vi "Periodic Tasks.vi"(8 "error in":errorcluster) -> ()   [LabVIEW 2015]
doc: "This VI runs in parallel to other tasks. It can contain as many user-defined periodic loops as you need. These can carry out PID or other sorts of timed response."
uses:
  <vilib>/Rock Robotics/WPI/Solenoid/WPI_SolenoidValue.ctl
  <vilib>/Rock Robotics/WPI/Utilities/WPI_GetSetVariantRefNum.vi
  <vilib>/Rock Robotics/WPI/Solenoid/WPI_SolenoidSetEnum.vi
  Robot Global Data.vi
  Vision/Vision Global.vi
  <vilib>/addons/control/pid/pid.llb/PID (DBL).vi
  <vilib>/addons/control/pid/NI_PID_pid.lvlib
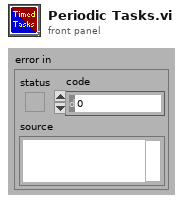
[diagram p1: front panel]
types:
  T1 = typedef "WPI_JoystickDevRef.ctl" = cluster{"Device":T2}
  T2 = typedef "WPI_JoystickDeviceEnum.ctl" = enum16{"USB 0", "USB 1", "USB 2", "USB 3", "USB 4", "USB 5"}
  T3 = typedef "WPI_MotorControlDeviceRef.ctl" = cluster{"DeviceStatus":errorcluster, "Type":T4, "PWM":cluster{"PWM Channel":T5, "DeadBand":T6}, "CAN":cluster{"Device Number":u8, "Control Mode":T7, "Semaphore":T8, "Max Vout":dbl, "TalonSRX Control Mode":T9}, "Invert":bool}
  T4 = typedef "WPI_MotorControlType.ctl" = enum16{"PWM", "CAN", "CANTalonSRX"}
  T5 = typedef "FPGA_DIOPWMChannel.ctl" = enum8{"PWM 0", "PWM 1", "PWM 2", "PWM 3", "PWM 4", "PWM 5", "PWM 6", "PWM 7", "PWM 8", "PWM 9", "PWM MXP 0", "PWM MXP 1", "PWM MXP 2", "PWM MXP 3", "PWM MXP 4", "PWM MXP 5", "PWM MXP 6", "PWM MXP 7", "PWM MXP 8", "PWM MXP 9", "Invalid"}
  T6 = typedef "WPI_PWMDeadband.ctl" = cluster{"Name":string, "maxPositivePwm":i32, "minPositivePwm":i32, "centerPwm":i32, "maxNegativePwm":i32, "minNegativePwm":i32, "angularRange":u16}
  T7 = typedef "WPI_CANJaguar_ControlMode.ctl" = enum8{"Percent VBus", "Current", "Speed", "Position", "Voltage"}
  T8 = typedef "Semaphore RefNum" = refnum<k1>
  T9 = typedef "WPI_CANTalonSRX_APIControlMode.ctl" = enum8{"Percent VBus", "Speed", "Position", "Slave", "Unchanged / Invalid", "Voltage Compensation", "Current", "Motion Profile"}
  T10 = cluster{"proportional gain (Kc)":dbl, "integral time (Ti, min)":dbl, "derivative time (Td, min)":dbl}
  T11 = cluster{"Distance (ft)":dbl, "Center":cluster{dbl, dbl}, "Normalized Rect":cluster{"Numeric":dbl, "Numeric 2":dbl, "Numeric 3":dbl, "Numeric 5":dbl}}[]
  T12 = cluster{"Distance (ft)":dbl, "Center":cluster{dbl, dbl}, "Normalized Rect":cluster{"Numeric":dbl, "Numeric 2":dbl, "Numeric 3":dbl, "Numeric 5":dbl}}
  T13 = typedef "WPI_SolenoidValue.ctl" = enum16{"Off", "On", "Forward", "Reverse"}
  T14 = typedef "WPI_SolenoidDevRef.ctl" = cluster{"DevStatus":errorcluster, "Pneumatics Control Module":u8, "Forward Solenoid Channel":T15, "Reverse Solenoid Channel":T15}
  T15 = typedef "WPI_SolenoidChannel.ctl" = enum8{"Solenoid 0", "Solenoid 1", "Solenoid 2", "Solenoid 3", "Solenoid 4", "Solenoid 5", "Solenoid 6", "Solenoid 7", "Invalid"}
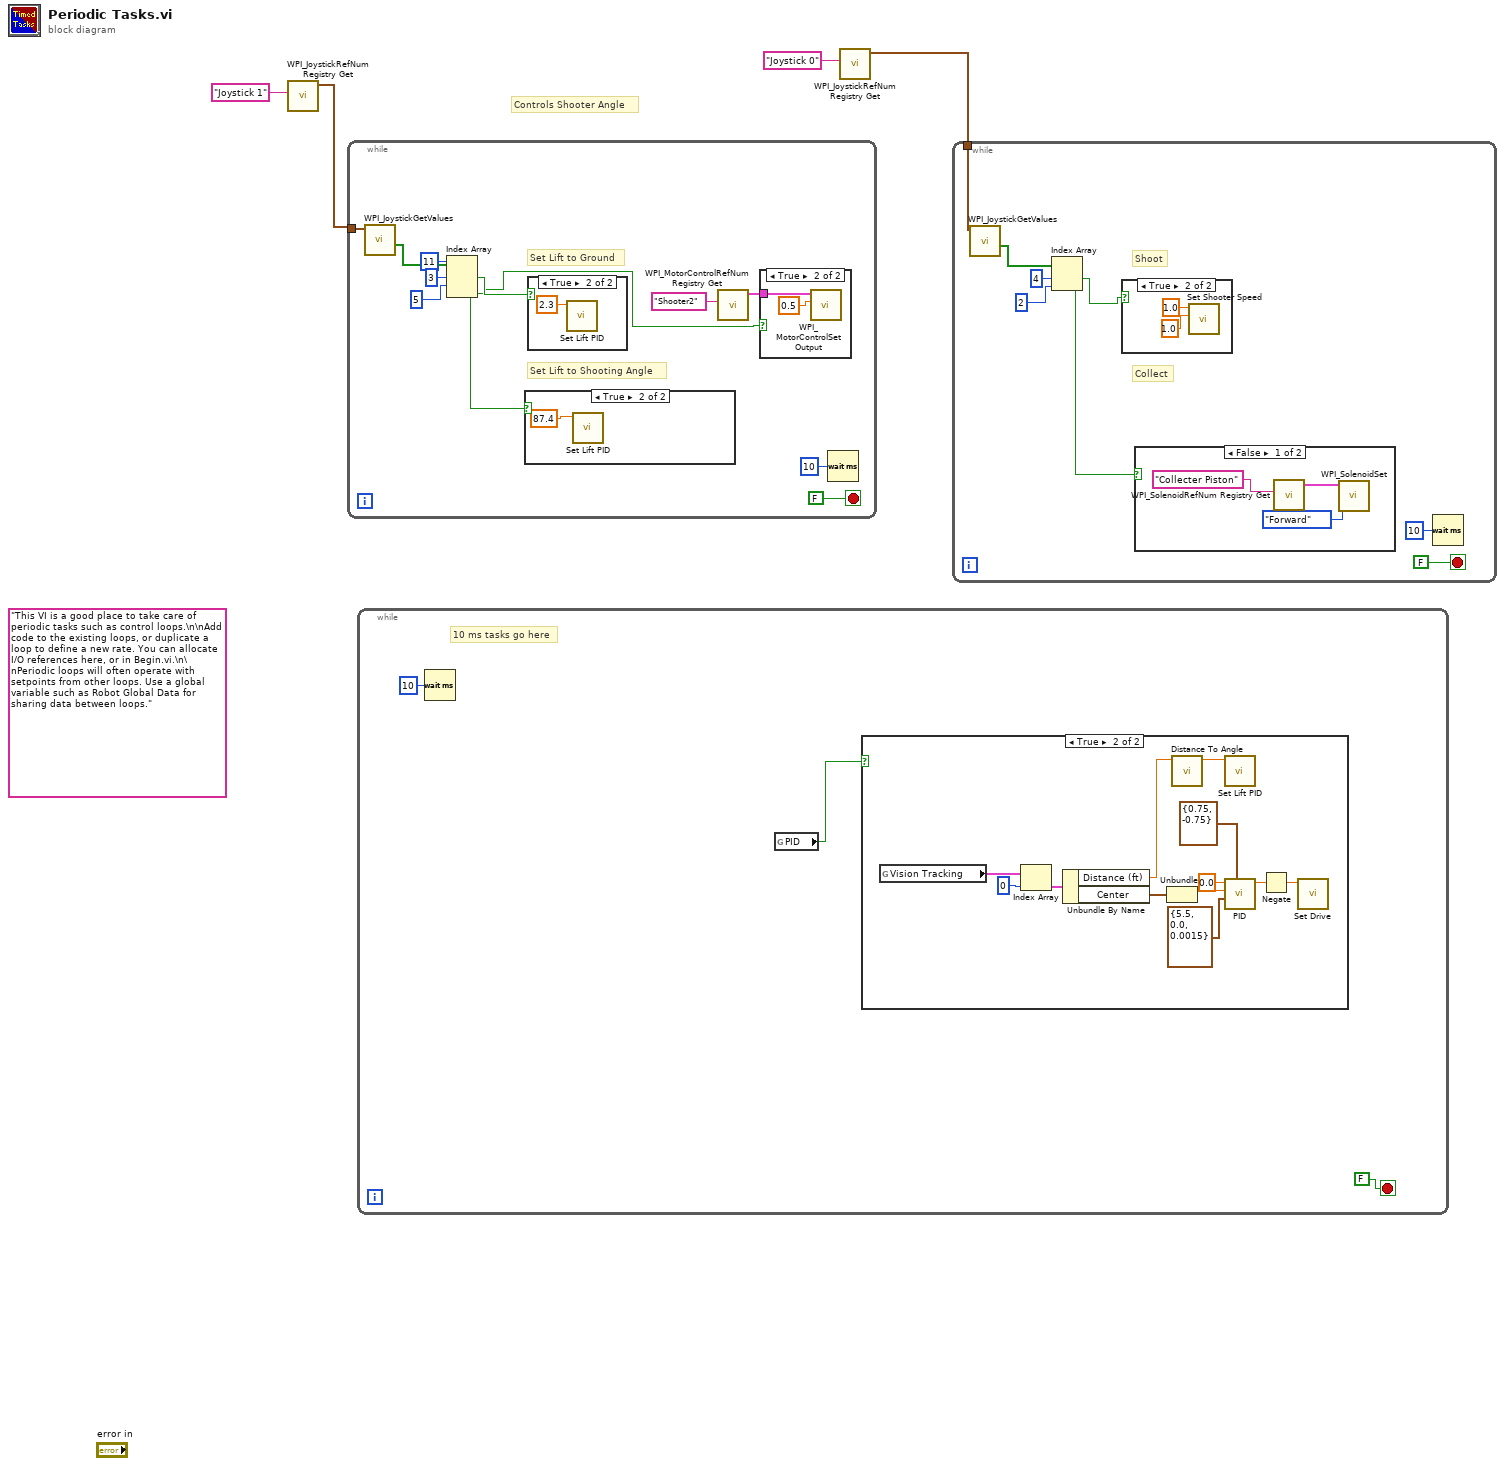
[diagram p0: block diagram]
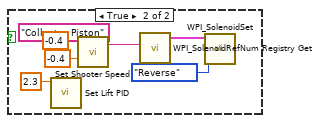
[diagram p2: hidden frame]
diagram:
  (unwired) "This VI is a good place to take care of periodic tasks such as control loops.\n\nAdd code to the existing loops, or duplicate a loop to define a new rate. You can allocate I/O references here, or in Begin.vi.\n\nPeriodic loops will often operate with setpoints from other loops. Use a global variable such as Robot Global Data for sharing data between loops."
  # "Controls Shooter Angle"
  n1 = call <vilib>:"WPI_JoystickRefNum Registry Get.vi"("refnum name"="Joystick 1") -> ("JoystickDevRef"=w3:T1)  [unwired: 1 in, 9 out]
  n2 = while {
    tunnel: w3 -> [w9]
    stop <- FALSE stop-if-true
    # "Set Lift to Shooting Angle"
    # "Set Lift to Ground"
    n3 = call <vilib>:"WPI_JoystickGetValues.vi"("JoystickDevRef"=w9) -> ("Buttons"=w14:bool[])  [unwired: 6 in, 4 out]
    n4 = Index Array(array=w14, index #1=3 ("index"), index #2=5 ("index"), index #3=11 ("index")) -> (element #1=w13:bool, element #2=w11:bool, element #3=w5:bool)
    n5 = case shown="True" w11 {
      frame False {
      }
      frame True {
        n6 = call "Set Lift PID.vi"("setpoint"=87.4) -> ()  [unwired: 11 in]
      }
    }
    n7 = case shown="True" w13 {
      frame False {
      }
      frame True {
        n8 = call "Set Lift PID.vi"("setpoint"=2.3) -> ()  [unwired: 11 in]
      }
    }
    n9 = call <vilib>:"WPI_MotorControlRefNum Registry Get.vi"("refnum name"="Shooter2" ("Motor 1")) -> ("MotorControlDevRef"=w7:T3)  [unwired: 9 in, 1 out]
    n10 = case shown="True" w5 {
      tunnel: w7 -> [_ w18]
      frame False {
      }
      frame True {
        n11 = call <vilib>:"WPI_MotorControlSetOutput.vi"("Output"=0.5, "MotorControlDevRef"=w18) -> ()  [unwired: 7 in, 3 out]
      }
    }
    n12 = Wait (ms)(milliseconds to wait=u32 10) -> ()  [unwired: 1 out]
  }
  n13 = while {
    stop <- FALSE stop-if-true
    # "10 ms tasks go here"
    n14 = Wait (ms)(milliseconds to wait=u32 10) -> ()  [unwired: 1 out]
    n15 = global read "Robot Global Data.vi" "PID"() -> (w21:bool)
    n16 = case shown="True" w21 {
      frame False {
      }
      frame True {
        n17 = global read "Vision Global.vi" "Vision Tracking"() -> (w33:T11)
        n18 = Index Array(array=w33, index=0) -> (element=w34:T12)
        n19 = Unbundle By Name(w34) -> ("Distance (ft)"=w27:dbl, "Center"=w32:cluster{dbl, dbl})
        n20 = Unbundle(w32) -> (w30:dbl)  [unwired: 1 out]
        n21 = call "Distance To Angle.vi"("Distance ft"=w27) -> ("Desired Angle"=w26:dbl)  [unwired: 10 in]
        n22 = call "Set Lift PID.vi"("setpoint"=w26) -> ()  [unwired: 11 in]
        n23 = call-poly <vilib>:"PID.vi"("output range"=cluster{"output high":dbl, "output low":dbl} {"output high"=0.75, "output low"=-0.75}, "PID gains"=T10 {"proportional gain (Kc)"=5.5, "integral time (Ti, min)"=0.0, "derivative time (Td, min)"=0.0015}, "process variable"=w30, "setpoint"=0.0) -> ("output"=w31:dbl)  [unwired: 6 in, 1 out]
        n24 = Negate(x=w31) -> (-x=w28:dbl)
        n25 = call "Set Drive.vi"("X axis value"=w28) -> ()  [unwired: 11 in]
      }
    }
  }
  n26 = call <vilib>:"WPI_JoystickRefNum Registry Get.vi"("refnum name"="Joystick 0") -> ("JoystickDevRef"=w1:T1)  [unwired: 1 in, 9 out]
  n27 = while {
    tunnel: w1 -> [w38]
    stop <- FALSE stop-if-true
    # "Collect"
    # "Shoot"
    n28 = call <vilib>:"WPI_JoystickGetValues.vi"("JoystickDevRef"=w38) -> ("Buttons"=w41:bool[])  [unwired: 6 in, 4 out]
    n29 = Index Array(array=w41, index #1=4 ("index"), index #2=2 ("index")) -> (element #1=w37:bool, element #2=w36:bool)
    n30 = case shown="True" w37 {
      frame False {
      }
      frame True {
        n31 = call "Set Shooter Speed.vi"("Set Bottom Speed"=1.0, "Set Top Speed"=1.0) -> ()  [unwired: 10 in]
      }
    }
    n32 = case shown="False" w36 {
      frame False {
        n33 = call <vilib>:"WPI_SolenoidRefNum Registry Get.vi"("refnum name"="Collecter Piston") -> ("SolenoidDevRef"=w45:T14)  [unwired: 9 in, 1 out]
        n34 = call-poly <vilib>:"WPI_SolenoidSet.vi"("Value"=WPI_SolenoidValue."Forward", "SolenoidDevRef"=w45) -> ()  [unwired: 8 in, 2 out]
      }
      frame True {
        n35 = call "Set Lift PID.vi"("setpoint"=2.3) -> ()  [unwired: 11 in]
        n36 = call "Set Shooter Speed.vi"("Set Bottom Speed"=-0.4, "Set Top Speed"=-0.4) -> ()  [unwired: 10 in]
        n37 = call <vilib>:"WPI_SolenoidRefNum Registry Get.vi"("refnum name"="Collecter Piston") -> ("SolenoidDevRef"=w48:T14)  [unwired: 9 in, 1 out]
        n38 = call-poly <vilib>:"WPI_SolenoidSet.vi"("Value"=WPI_SolenoidValue."Reverse", "SolenoidDevRef"=w48) -> ()  [unwired: 8 in, 2 out]
      }
    }
    n39 = Wait (ms)(milliseconds to wait=u32 10) -> ()  [unwired: 1 out]
  }
